vi "RemoveNode.vi"(8 "error in (no error)":errorcluster, 10 "Node ref":refnum<data-value>, 11 "DirectedGraphWorldMap in":refnum<class "NI_Robotics_DirectedGraphWorldMap.lvclass">) -> (0 "error out":errorcluster, 3 "DirectedGraphWorldMap out":refnum<class "NI_Robotics_DirectedGraphWorldMap.lvclass">)   [LabVIEW 2017, in "NI_Robotics_DirectedGraphWorldMap.lvclass"]
uses:
  <vilib>/robotics/Navigation/shared/WorldMap/DirectedGraphWorldMap/NI_Robotics_DirectedGraphWorldMap.lvclass
  <vilib>/robotics/Navigation/shared/MapNode/AbstractMapNode/NI_Robotics_AbstractMapNode.lvclass
  <vilib>/robotics/Navigation/shared/MapNode/DirectedGraphMapNode/NI_Robotics_DirectedGraphMapNode.lvclass
  c:/Program Files (x86)/National Instruments/LabVIEW 2017/vi.lib/robotics/Navigation/shared/MapNode/AbstractDstarNode/NI_Robotics_AbstractDstarNode.lvclass
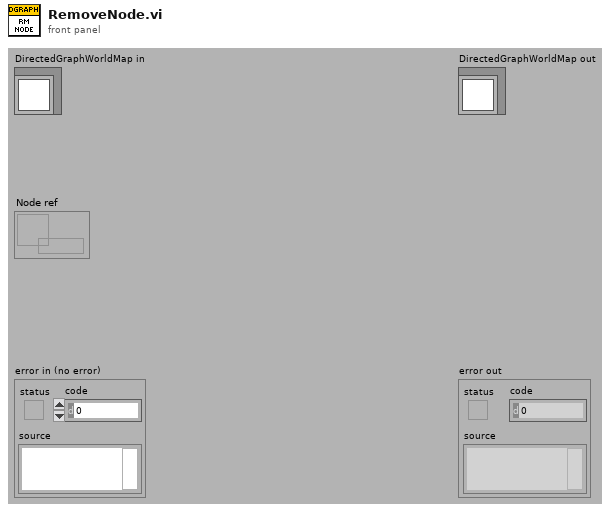
[diagram p1: front panel]
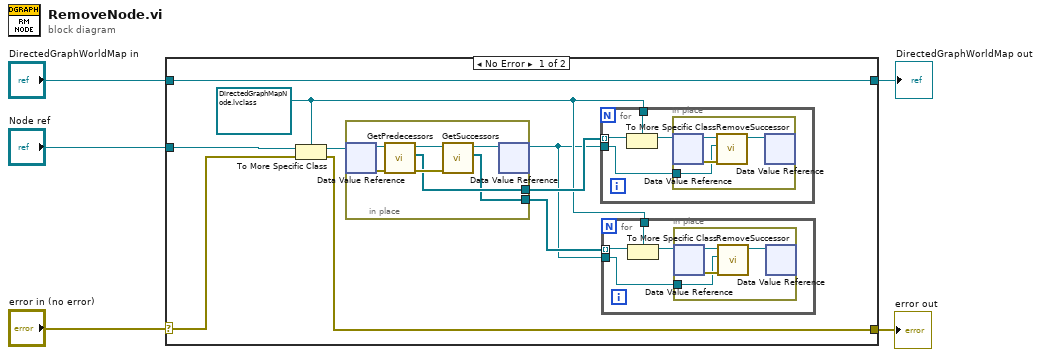
[diagram p0: block diagram]
diagram:
  n1 = case shown="No Error" "error in (no error)" {
    selector: "error in (no error)" -> [w12 w39]
    tunnel: [w14 w39] -> w4
    tunnel: [w13 w38] -> w2
    tunnel: "DirectedGraphWorldMap in" -> [w13 w38]
    tunnel: "Node ref" -> [w11 _]
    frame No Error {
      w8 = refnum<data-value> refnum ("Node Ref")
      n2 = To More Specific Class(target class=w8, reference=w11, error in=w12) -> (specific class reference=w10:refnum<data-value>, error out=w14:errorcluster)
      n3 = in-place {
        in-place-border: [w32] -> w9
        in-place-border: [w31] -> w7
        n4 = in-place-dvr #1(w10) -> (w36:refnum<class "NI_Robotics_DirectedGraphMapNode.lvclass">, w37:errorcluster)
        n5 = call-dynamic "GetPredecessors.vi"("error in (no error)"=w37, "DirectedGraphMapNode in"=w36) -> ("error out"=w33:errorcluster, "Predecessors"=w32:refnum<data-value>[], "DirectedGraphMapNode out"=w35:refnum<class "NI_Robotics_DirectedGraphMapNode.lvclass">)  [unwired: 6 in, 1 out]
        n6 = call-dynamic "GetSuccessors.vi"("error in (no error)"=w33, "DirectedGraphMapNode in"=w35) -> ("Successors"=w31:refnum<data-value>[], "DirectedGraphMapNode out"=w34:refnum<class "NI_Robotics_DirectedGraphMapNode.lvclass">)  [unwired: 6 in, 2 out]
        n7 = in-place-dvr #1(w34) -> (w6:refnum<data-value>)  [unwired: 1 out]
      }
      n8 = for {
        tunnel: w9 -> [w25] mode=indexing
        tunnel: w6 -> [w26]
        tunnel: w8 -> [w24]
        n9 = To More Specific Class(target class=w24, reference=w25) -> (specific class reference=w23:refnum<data-value>)  [unwired: 1 in, 1 out]
        n10 = in-place {
          in-place-border: w26 -> [w27]
          n11 = in-place-dvr #2(w23) -> (w30:refnum<class "NI_Robotics_DirectedGraphMapNode.lvclass">, w28:errorcluster)
          n12 = call-dynamic "RemoveSuccessor.vi"("error in (no error)"=w28, "Node Ref"=w27, "DirectedGraphMapNode in"=w30) -> ("DirectedGraphMapNode out"=w29:refnum<class "NI_Robotics_DirectedGraphMapNode.lvclass">)  [unwired: 7 in, 1 out]
          n13 = in-place-dvr #2(w29) -> ()  [unwired: 2 out]
        }
      }
      n14 = for {
        tunnel: w7 -> [w17] mode=indexing
        tunnel: w6 -> [w18]
        tunnel: w8 -> [w16]
        n15 = To More Specific Class(target class=w16, reference=w17) -> (specific class reference=w15:refnum<data-value>)  [unwired: 1 in, 1 out]
        n16 = in-place {
          in-place-border: w18 -> [w19]
          n17 = in-place-dvr #3(w15) -> (w22:refnum<class "NI_Robotics_DirectedGraphMapNode.lvclass">, w20:errorcluster)
          n18 = call-dynamic "RemoveSuccessor.vi"("error in (no error)"=w20, "Node Ref"=w19, "DirectedGraphMapNode in"=w22) -> ("DirectedGraphMapNode out"=w21:refnum<class "NI_Robotics_DirectedGraphMapNode.lvclass">)  [unwired: 7 in, 1 out]
          n19 = in-place-dvr #3(w21) -> ()  [unwired: 2 out]
        }
      }
    }
    frame Error {
    }
  }
  "error out" <- w4
  "DirectedGraphWorldMap out" <- w2
